vi "Vanna Control Loop.vi"() -> ()   [LabVIEW 2019]
uses:
  <vilib>/Rock Robotics/WPI/ThirdParty/Phoenix-LabVIEW/Motor Controller/Controls/CTRE_Phoenix_MotorControl_ControlMode.ctl
  Calculations or utilities/Is command done typedef.ctl
  Vanna Global.vi
  <vilib>/Rock Robotics/WPI/Solenoid/WPI_SolenoidValue.ctl
  <vilib>/Rock Robotics/WPI/Solenoid/WPI_SolenoidSetEnum.vi
  <vilib>/Rock Robotics/Network Tables/NT Write Number.vi
  <vilib>/Rock Robotics/Network Tables/NT Write String.vi
  .Team Code/Robot Global Data.vi
panel:
  out "Proximity":u16
  out "Normalized Color":cluster{"R":dbl, "G":dbl, "B":dbl}
  out "Confidence":dbl
  out "Matched Color Name":string
  out "Color":u32(colorbox)
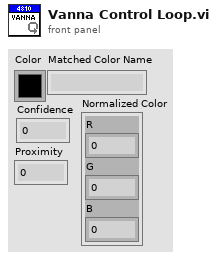
[diagram p1: front panel]
types:
  T1 = typedef "WPI_MotorControlDeviceRef.ctl" = cluster{"DeviceStatus":errorcluster, "Type":T2, "PWM":cluster{"PWM Channel":T3, "DeadBand":T4}, "CAN":cluster{"Device Number":u8, "SetOutput VI Ref":variant, "GetOutput VI Ref":variant, "Enable VI Ref":variant, "Disable VI Ref":variant, "Data":variant}, "Invert":bool, "DIO PWM":cluster{"PWM \"Enable\" Channel":T3, "DIOChannel":T5, "PWM Rate":dbl}}
  T2 = typedef "WPI_MotorControlType.ctl" = enum16{"PWM", "CAN", "DIO PWM"}
  T3 = typedef "FPGA_DIOPWMChannel.ctl" = enum8{"PWM 0", "PWM 1", "PWM 2", "PWM 3", "PWM 4", "PWM 5", "PWM 6", "PWM 7", "PWM 8", "PWM 9", "PWM MXP 0", "PWM MXP 1", "PWM MXP 2", "PWM MXP 3", "PWM MXP 4", "PWM MXP 5", "PWM MXP 6", "PWM MXP 7", "PWM MXP 8", "PWM MXP 9", "Invalid"}
  T4 = typedef "WPI_PWMDeadband.ctl" = cluster{"Name":string, "maxPositivePwm":i32, "minPositivePwm":i32, "centerPwm":i32, "maxNegativePwm":i32, "minNegativePwm":i32, "angularRange":u16}
  T5 = typedef "FPGA_DIOChannel.ctl" = enum8{"DIO 0", "DIO 1", "DIO 2", "DIO 3", "DIO 4", "DIO 5", "DIO 6", "DIO 7", "DIO 8", "DIO 9", "DIO MXP 0", "DIO MXP 1", "DIO MXP 2", "DIO MXP 3", "DIO MXP 4", "DIO MXP 5", "DIO MXP 6", "DIO MXP 7", "DIO MXP 8", "DIO MXP 9", "DIO MXP 10", "DIO MXP 11", "DIO MXP 12", "DIO MXP 13", "DIO MXP 14", "DIO MXP 15", "SPI Port CS1", "SPI Port CS2", "SPI Port CS3", "SPI Port MISO", "SPI Port MOSI", "Invalid"}
  T6 = typedef "WPI_SolenoidDevRef.ctl" = cluster{"DevStatus":errorcluster, "Pneumatics Control Module":u8, "Forward Solenoid Channel":T7, "Reverse Solenoid Channel":T7}
  T7 = typedef "WPI_SolenoidChannel.ctl" = enum8{"Solenoid 0", "Solenoid 1", "Solenoid 2", "Solenoid 3", "Solenoid 4", "Solenoid 5", "Solenoid 6", "Solenoid 7", "Invalid"}
  T8 = typedef "Color Sensor V3 DevRef.ctl" = cluster{"I2CDevRef":T9}
  T9 = typedef "WPI_I2CDevRef.ctl" = cluster{"DevStatus":errorcluster, "Device Address":u8, "Handle":i32, "I2C Bus":T10}
  T10 = typedef "i2c_bus.ctl" = enum16{"I2C On-Board", "I2C MXP", "Invalid"}
  T11 = typedef "Is command done typedef.ctl" = cluster{"Done?":bool, "Timestamp [ms]":dbl}
  T12 = typedef "WPI_SolenoidValue.ctl" = enum16{"Off", "On", "Forward", "Reverse"}
  T13 = typedef "Vanna Command Type Def.ctl" = cluster{"Vanna Mode":T14, "Throttle (%)":dbl, "Timestamp (ms)":dbl}
  T14 = typedef "Vanna Mode Type Def.ctl" = enum16{"Disabled", "Raw Throttle", "Rotation Control", "Position Control"}
  T15 = typedef "CTRE_Phoenix_MotorControl_ControlMode.ctl" = u16
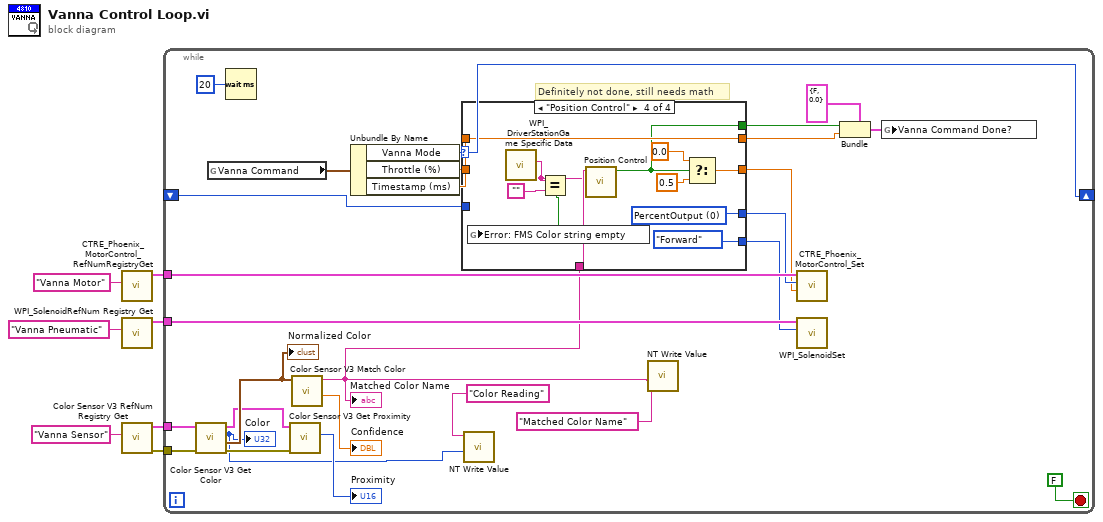
[diagram p0: block diagram]
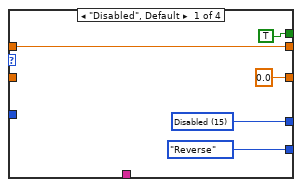
[diagram p2: hidden frame]
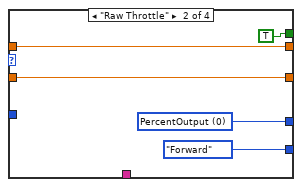
[diagram p3: hidden frame]
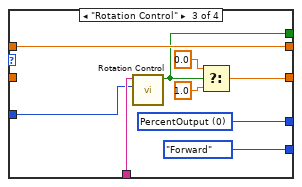
[diagram p4: hidden frame]
diagram:
  n1 = call <vilib>:"CTRE_Phoenix_MotorControl_RefNumRegistryGet.vi"("refnum name"="Vanna Motor") -> ("PhoenixMotorControlDevRef"=w6:T1)  [unwired: 9 in, 1 out]
  n2 = call <vilib>:"WPI_SolenoidRefNum Registry Get.vi"("refnum name"="Vanna Pneumatic") -> ("SolenoidDevRef"=w4:T6)  [unwired: 9 in, 1 out]
  n3 = call <vilib>:"Color Sensor V3 RefNum Registry Get.vi"("refnum name"="Vanna Sensor") -> ("error out"=w1:errorcluster, "ColorSensorDevRef"=w2:T8)  [unwired: 9 in]
  n4 = while {
    tunnel: w6 -> [w32]
    tunnel: w4 -> [w22]
    tunnel: w2 -> [w20]
    tunnel: w1 -> [w15]
    shift-right: [w9] -> _
    shift-left: _ -> [w8]
    stop <- FALSE stop-if-true
    # "Definitely not done, still needs math"
    n5 = call <vilib>:"Color Sensor V3 Get Color.vi"("error in (no error)"=w15, "ColorSensorDevRef"=w20) -> ("error out"=w14:errorcluster, "Normalized Color"=w19:cluster{"R":dbl, "G":dbl, "B":dbl}, "Color"=w13:u32, "ColorSensorDevRef out"=w18:T8)  [unwired: 6 in]
    "Color" <- w13
    "Normalized Color" <- w19
    n6 = global read "Vanna Global.vi" "Vanna Command"() -> (w25:T13)
    n7 = Wait (ms)(milliseconds to wait=u32 20) -> ()  [unwired: 1 out]
    n8 = call <vilib>:"Color Sensor V3 Get Proximity.vi"("error in (no error)"=w14, "ColorSensorDevRef"=w18) -> ("Proximity"=→"Proximity":u16)  [unwired: 7 in, 2 out]
    n9 = call <vilib>:"Color Sensor V3 Match Color.vi"("Measured Color"=w19) -> ("Confidence"=→"Confidence":dbl, "Matched Color Name"=w10:string)  [unwired: 8 in, 1 out]
    "Matched Color Name" <- w10
    n10 = Unbundle By Name(w25) -> ("Vanna Mode"=w9:T14, "Throttle (%)"=w31:dbl, "Timestamp (ms)"=w30:dbl)
    n11 = case shown="\"Position Control\"" w9 {
      tunnel: w31 -> [_ w41 _ _]
      tunnel: w30 -> [w39 w44 w53 w63]
      tunnel: [w39 w44 w53 w63] -> w27
      tunnel: [w38 w43 w52 w64] -> w29
      tunnel: [TRUE ("Done?") TRUE ("Done?") w51 w62] -> w26
      tunnel: [0.0 ("Throttle (%)") w41 w48 w59] -> w23
      tunnel: [WPI_SolenoidValue."Reverse" ("Value") WPI_SolenoidValue."Forward" ("Value") WPI_SolenoidValue."Forward" ("Value") WPI_SolenoidValue."Forward" ("Value")] -> w21
      tunnel: w10 -> [_ _ w46 w57]
      tunnel: w8 -> [_ _ w45 _]
      frame "Disabled", Default {
        w38 = T15 15 items=["PercentOutput"=0, "Position"=1, "Velocity"=2, "Current"=3, "Follower"=5, "MotionProfile"=6, "MotionMagic"=7, "MotionProfileArc"=10, "Disabled"=15] ("Control Mode")
      }
      frame "Raw Throttle" {
        w43 = T15 0 items=["PercentOutput"=0, "Position"=1, "Velocity"=2, "Current"=3, "Follower"=5, "MotionProfile"=6, "MotionMagic"=7, "MotionProfileArc"=10, "Disabled"=15] ("Control Mode")
      }
      frame "Rotation Control" {
        w52 = T15 0 items=["PercentOutput"=0, "Position"=1, "Velocity"=2, "Current"=3, "Follower"=5, "MotionProfile"=6, "MotionMagic"=7, "MotionProfileArc"=10, "Disabled"=15] ("Control Mode")
        n12 = call "Rotation Control.vi"("Prior Mode"=w45, "Color Sensor Input"=w46) -> ("Done"=w51:bool)  [unwired: 9 in]
        n13 = Select(t=0.0, s=w51, f=1.0) -> (s? t:f=w48:dbl)
      }
      frame "Position Control" {
        w64 = T15 0 items=["PercentOutput"=0, "Position"=1, "Velocity"=2, "Current"=3, "Follower"=5, "MotionProfile"=6, "MotionMagic"=7, "MotionProfileArc"=10, "Disabled"=15] ("Control Mode")
        n14 = call <vilib>:"WPI_DriverStationGame Specific Data.vi"() -> ("Game Specific Data"=w54:string)  [unwired: 11 in]
        n15 = Equal?(x=w54, y="") -> (x = y?=w55:bool)
        n16 = global write "Robot Global Data.vi" "Error: FMS Color string empty"(w55) -> ()
        n17 = call "Position Control.vi"("FMS Desired Color"=w54, "Color Sensor Input"=w57) -> ("Are we done?"=w62:bool)  [unwired: 9 in]
        n18 = Select(t=0.0, s=w62, f=0.5) -> (s? t:f=w59:dbl)
      }
    }
    n19 = call-poly <vilib>:"NT Write Value.vi"("Numeric"=w13, "Name"="Color Reading") -> ()  [unwired: 9 in, 1 out]
    n20 = call-poly <vilib>:"NT Write Value.vi"("String"=w10, "Name"="Matched Color Name") -> ()  [unwired: 9 in, 1 out]
    n21 = call <vilib>:"CTRE_Phoenix_MotorControl_Set.vi"("Output"=w23, "Control Mode"=w29, "PhoenixMotorControlDevRef"=w32) -> ()  [unwired: 7 in, 2 out]
    n22 = call-poly <vilib>:"WPI_SolenoidSet.vi"("Value"=w21, "SolenoidDevRef"=w22) -> ()  [unwired: 8 in, 2 out]
    n23 = Bundle(cluster=T11 {"Done?"=FALSE, "Timestamp [ms]"=0.0} ("Command Done?"), "Done?"=w26, "Timestamp [ms]"=w27) -> (w24:T11)
    n24 = global write "Vanna Global.vi" "Vanna Command Done?"(w24) -> ()
  }
